vi "ryerror_unpack.vi"(8 "error in (no error)":errorcluster, 9 "message in":string) -> (0 "error out":errorcluster)   [LabVIEW 2017]
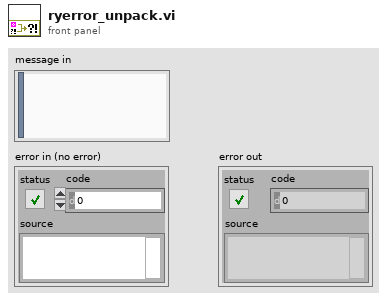
[diagram p1: front panel]
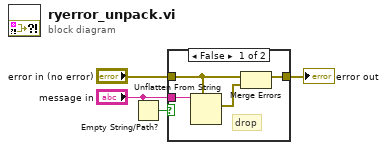
[diagram p0: block diagram]
diagram:
  n1 = Empty String/Path?(string/path="message in") -> (empty?=w1:bool)
  n2 = case shown="False" w1 {
    tunnel: "message in" -> [w8 _]
    tunnel: "error in (no error)" -> [w7 w9]
    tunnel: [w5 w9] -> w3
    frame False {
      # "drop"
      n3 = Unflatten From String(type=w7, binary string=w8) -> (value=w6:errorcluster)  [unwired: 3 in, 2 out]
      n4 = Merge Errors(w7, w6) -> (w5:errorcluster)
    }
    frame True {
    }
  }
  "error out" <- w3
